vi "Read 1D Strings From Config.vi"(11 "key":string) -> (3 "1D array strings":string[](array[string]))   [LabVIEW 2020, in "Text-Based VI Icon.lvlib"]
uses:
  Text-Based VI Icon.lvlib
  <resource>/dialog/lvconfig.llb/LV Config Read String.vi
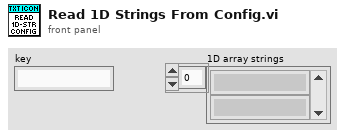
[diagram p1: front panel]
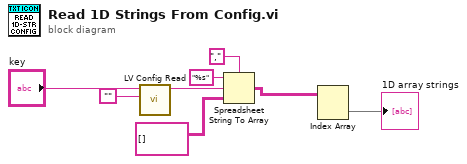
[diagram p0: block diagram]
diagram:
  n1 = call-poly <resource>:"LV Config Read.vi"("default value"="", "key"="key") -> ("value"=w5:string)  [unwired: 3 in, 2 out]
  n2 = Spreadsheet String To Array(delimiter (Tab)=",", format string="%s", spreadsheet string=w5, array type (2D Dbl)=string[][] []) -> (array=w2:string[][])
  n3 = Index Array(array=w2) -> (element=→"1D array strings":string[])  [unwired: 2 in]
